vi "DRAM Pack data-test.vi"() -> ()   [LabVIEW 2015]
panel:
  out "output":bool=TRUE
  in  "Input valid?":bool=TRUE
  in  "Elements to write":i32
  out "Array":u32[](array[numeric])
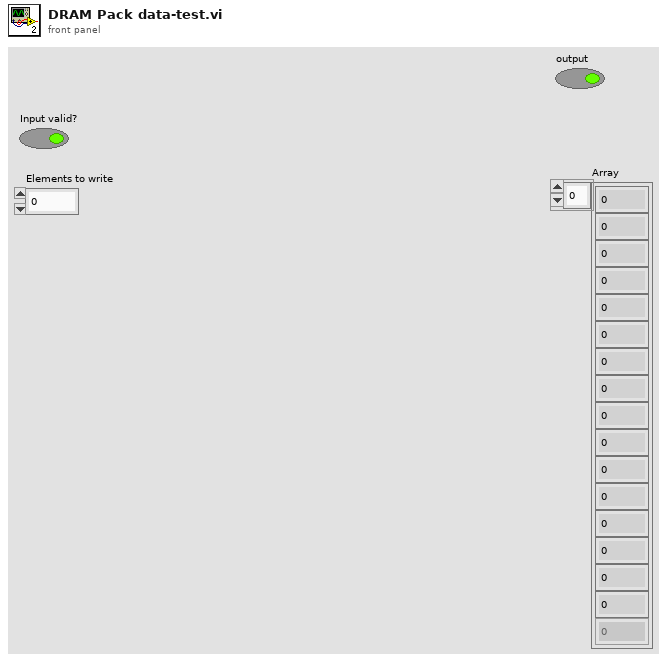
[diagram p1: front panel]
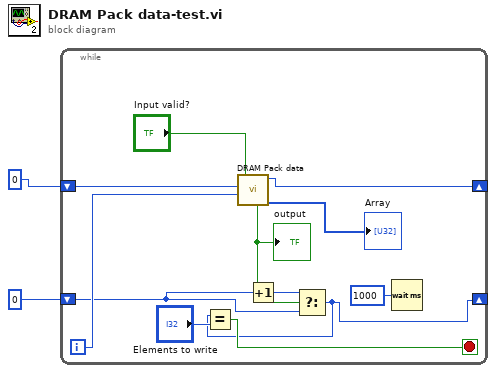
[diagram p0: block diagram]
diagram:
  n1 = while {
    shift-right: [w12] -> _
    shift-left: u32 0 ("Adress input") -> [w13]
    shift-right: [w3] -> _
    shift-left: u32 0 ("Adress input") -> [w6]
    i -> [w9]
    stop <- w4 stop-if-true
    n2 = call "DRAM Pack data.vi"("Data input"=w9, "Adress input"=w13, "Input valid?"="Input valid?") -> ("Array"=→"Array":u32[], "Address output"=w12:u32, "output"=w7:bool)  [unwired: 6 in]
    "output" <- w7
    n3 = Increment(x=w6) -> (x+1=w5:u32)
    n4 = Select(t=w5, s=w7, f=w6) -> (s? t:f=w3:u32)
    n5 = Equal?(x=w3, y="Elements to write") -> (x = y?=w4:bool)
    n6 = Wait (ms)(milliseconds to wait=u32 1000) -> ()  [unwired: 1 out]
  }
